vi "SRV_SRV_zZ Notifier.vi"(6 "Notifier Methods":T1, 8 "error in (no error)":errorcluster, 9 "timeout in ms (-1)":i32, 10 "Notification String":string) -> (0 "error out":errorcluster)   [LabVIEW 2014]
doc: "Manges the \"SRV_Loops\" notifier used for some of the synchronization between the two loops.\n\n\nAuthor: Mike Schultz - Logic PD"
uses:
  SRV_SRV_Loops Notifier Methods.ctl
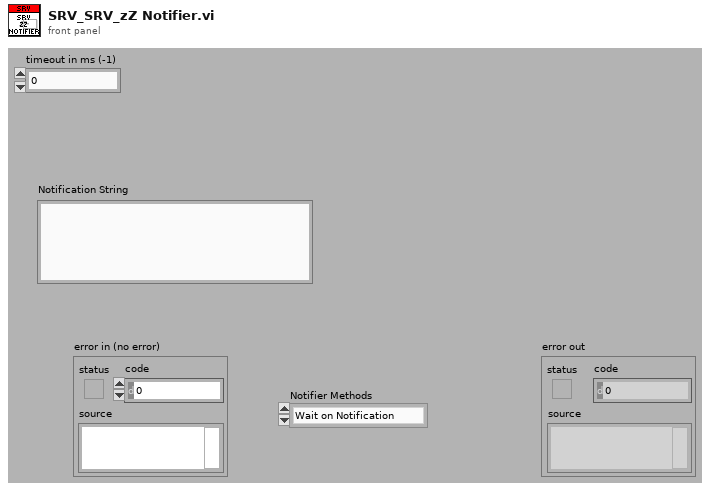
[diagram p1: front panel]
types:
  T1 = typedef "SRV_SRV_Loops Notifier Methods.ctl" = enum16{"Wait on Notification", "Send Notification", "Release Notifier"}
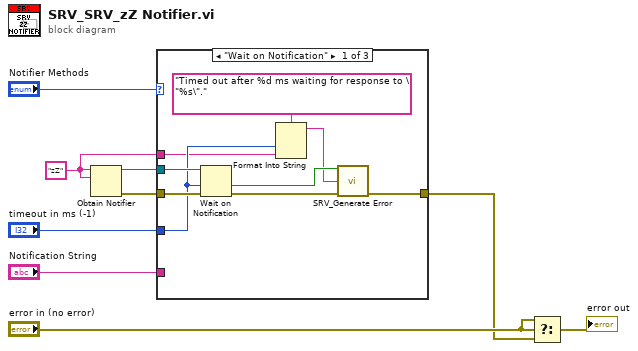
[diagram p0: block diagram]
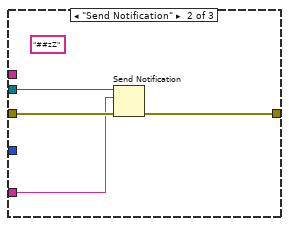
[diagram p2: hidden frame]
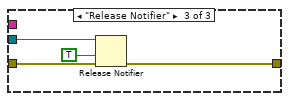
[diagram p3: hidden frame]
diagram:
  w1 = "zZ" ("name (unnamed)")
  n1 = Obtain Notifier(name (unnamed)=w1, notification data type=w1) -> (notifier out=w6:refnum<notifier>, error out=w5:errorcluster)  [unwired: 2 in, 1 out]
  n2 = case shown="\"Wait on Notification\"" "Notifier Methods" {
    tunnel: [w15 w22 w26] -> w7
    tunnel: w6 -> [w17 w21 w24]
    tunnel: w5 -> [w18 w20 w25]
    tunnel: "Notification String" -> [_ w19 _]
    tunnel: "timeout in ms (-1)" -> [w11 _ _]
    tunnel: w1 -> [w10 _ _]
    frame "Wait on Notification" {
      n3 = Wait on Notification(notifier=w17, timeout in ms (-1)=w11, error in (no error)=w18) -> (timed out?=w14:bool, error out=w16:errorcluster)  [unwired: 1 in, 2 out]
      n4 = Format Into String(format string="Timed out after %d ms waiting for response to \"%s\".", w11, w10) -> (resulting string=w13:string)  [unwired: 2 in, 1 out]
      n5 = call "SRV_Generate Error.vi"("status (T)"=w14, "Message"=w13, "error in (no error)"=w16) -> ("error out"=w15:errorcluster)  [unwired: 12 in]
    }
    frame "Send Notification" {
      (unwired) "##zZ" ("notification")
      n6 = Send Notification(notification=w19, notifier=w21, error in (no error)=w20) -> (error out=w22:errorcluster)  [unwired: 1 out]
    }
    frame "Release Notifier" {
      n7 = Release Notifier(notifier=w24, force destroy? (F)=TRUE, error in (no error)=w25) -> (error out=w26:errorcluster)  [unwired: 2 out]
    }
  }
  n8 = Select(t="error in (no error)", s="error in (no error)", f=w7) -> (s? t:f=→"error out":errorcluster)
